vi "MeasurementItems_DeleteChannels.vi"(8 "error in (no error)":errorcluster, 10 "# Channel":i32[](array[numeric]), 11 "OXY_SCPI Reseource In":refnum<visa-resource-name>) -> (0 "error out":errorcluster, 1 "communication_data":T1, 3 "OXY_SCPI Reseource Out":refnum<visa-resource-name>)   [LabVIEW 2018, in "OXYGEN.lvlib"]
doc: "Delete Items, shift remaining to left."
uses:
  OXYGEN.lvlib
  TypeDefs/Cluster_RawCommData.ctl
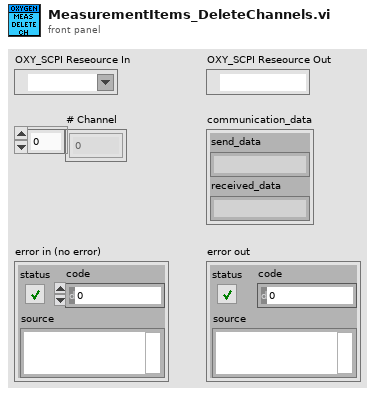
[diagram p1: front panel]
types:
  T1 = typedef "OXYGEN.lvlib/Cluster_RawCommData.ctl" = cluster{"send_data":string, "received_data":string}
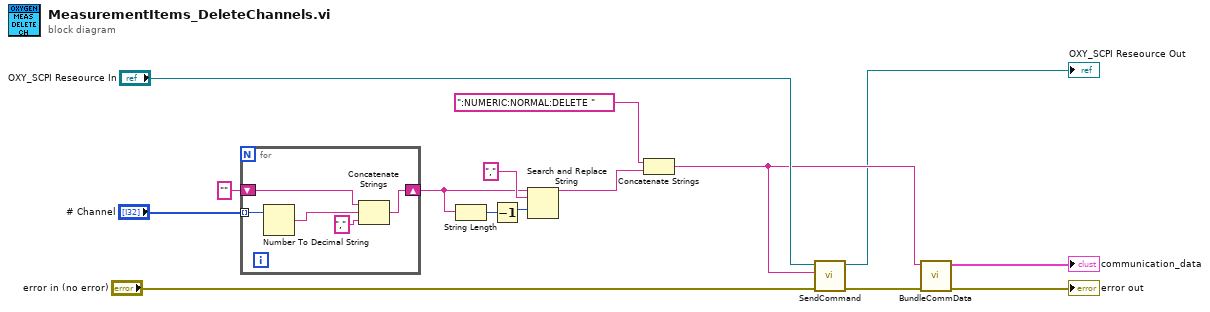
[diagram p0: block diagram]
diagram:
  n1 = for {
    tunnel: "# Channel" -> [w18] mode=indexing
    shift-right: [w19] -> w8
    shift-left: "" -> [w16]
    n2 = Number To Decimal String(number=w18) -> (decimal integer string=w17:string)  [unwired: 1 in]
    n3 = Concatenate Strings(w16, w17, "," ("string")) -> (w19:string)
  }
  n4 = String Length(string=w8) -> (length=w7:i32)
  n5 = Decrement(x=w7) -> (x-1=w10:i32)
  n6 = Search and Replace String(input string=w8, search string=",", offset=w10) -> (result string=w1:string)  [unwired: 5 in, 3 out]
  n7 = Concatenate Strings(":NUMERIC:NORMAL:DELETE " ("t"), w1) -> (w4:string)
  n8 = call "SendCommand.vi"("error in (no error)"="error in (no error)", "String to Send"=w4, "OXY_SCPI Reseource In"="OXY_SCPI Reseource In") -> ("error out"=w3:errorcluster, "OXY_SCPI Reseource Out"=→"OXY_SCPI Reseource Out":refnum<visa-resource-name>)  [unwired: 7 in]
  n9 = call "BundleCommData.vi"("error in (no error)"=w3, "send_data"=w4) -> ("error out"=→"error out":errorcluster, "communication_data"=→"communication_data":T1)  [unwired: 8 in]
